vi "Team Colors.vi"() -> (2 "Team Colors":u32[](array[colorbox])=[6618880, 16711680, 255, 16776960, 16711935, 65535, 16744448, 8421631, 16711808, 16448250])   [LabVIEW 2020, in "SquareBattle.lvlib"]
uses:
  SquareBattle.lvlib
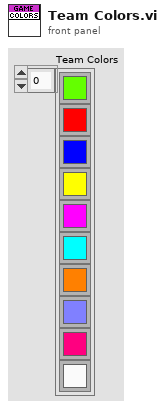
[diagram p1: front panel]
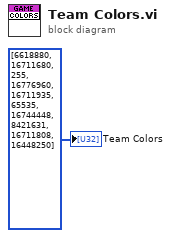
[diagram p0: block diagram]
diagram:
  "Team Colors" <- u32[] [6618880, 16711680, 255, 16776960, 16711935, 65535, 16744448, 8421631, 16711808, 16448250]
